vi "is_collection_exist.vi"(0 "abstract_vector_base in":refnum<class "abstract_vector_base.lvclass">, 5 "collection_name":string, 11 "error in (no error)":errorcluster) -> (4 "abstract_vector_base out":refnum<class "abstract_vector_base.lvclass">, 6 "exist? (True: Exist)":bool, 15 "error out":errorcluster)   [LabVIEW 2020, in "abstract_vector_base.lvclass"]
uses:
  abstract_vector_base.lvclass
  820372bd-fc1d-49d9-a77d-5c69df4709bd.vi
  <vilib>/Comparison/Equal/Equal Functor/Equal Functor.lvclass
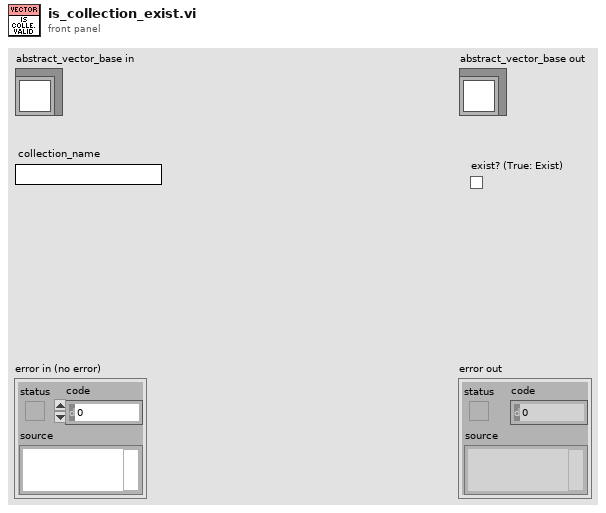
[diagram p1: front panel]
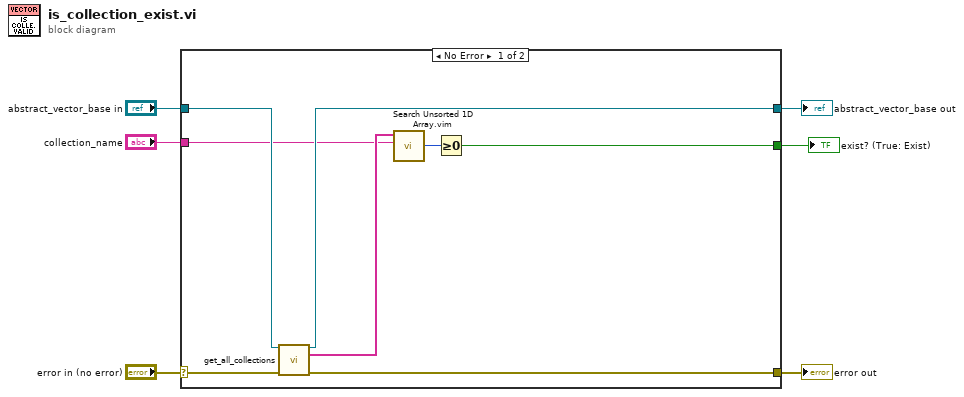
[diagram p0: block diagram]
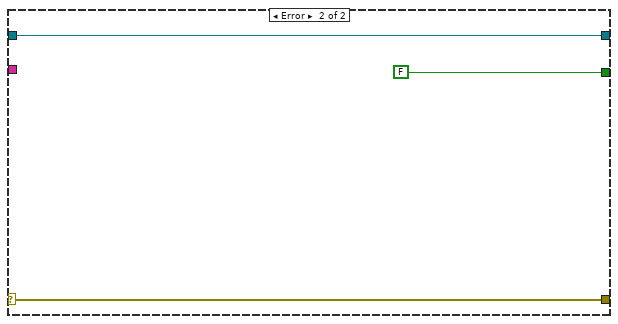
[diagram p2: hidden frame]
diagram:
  n1 = case shown="No Error" "error in (no error)" {
    selector: "error in (no error)" -> [w13 w17]
    tunnel: [w12 w17] -> w5
    tunnel: [w11 w16] -> w3
    tunnel: "abstract_vector_base in" -> [w14 w16]
    tunnel: "collection_name" -> [w9 _]
    tunnel: [w7 FALSE] -> w1
    frame No Error {
      n2 = call-dynamic "get_all_collections.vi"("abstract_vector_base in"=w14, "error in (no error)"=w13) -> ("abstract_vector_base out"=w11:refnum<class "abstract_vector_base.lvclass">, "collection"=w10:string[], "error out"=w12:errorcluster)  [unwired: 11 in]
      n3 = call "Search Unsorted 1D Array.vim"("element"=w9, "unsorted 1D array"=w10) -> ("index of element"=w8:i32)  [unwired: 9 in]
      n4 = Greater Or Equal To 0?(x=w8) -> (x >= 0?=w7:bool)
    }
    frame Error {
    }
  }
  "error out" <- w5
  "abstract_vector_base out" <- w3
  "exist? (True: Exist)" <- w1
